vi "PT 100 Spannung zu Temp (SubVI).vi"(2 "Temp PT 100 soll":dbl, 3 "U ist 2":fxp<+/-,16,4>) -> (0 "U soll":fxp<+/-,16,4> format="%.14g", 1 "Temp PT 100 ist":dbl)   [LabVIEW 2010]
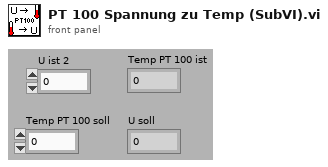
[diagram p1: front panel]
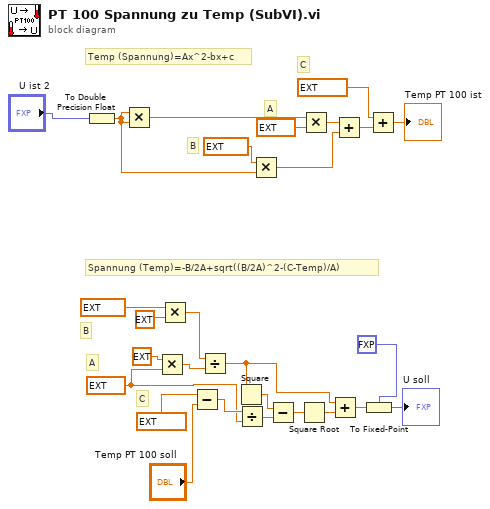
[diagram p0: block diagram]
diagram:
  w6 = ext 2.1471000000000000001 ("y")
  # "C"
  # "A"
  # "B"
  # "Spannung (Temp)=-B/2A+sqrt((B/2A)^2-(C-Temp)/A)"
  # "Temp (Spannung)=Ax^2-bx+c"
  # "C"
  # "A"
  # "B"
  n1 = To Double Precision Float(number="U ist 2") -> (double precision float=w1:dbl)
  n2 = Multiply(x=w1, y=w1) -> (x*y=w27:dbl)
  n3 = Multiply(x=ext 2.0 ("y"), y=w6) -> (x*y=w15:ext)
  n4 = Multiply(x=ext 111.873 ("y"), y=ext -1.0) -> (x*y=w17:ext)
  n5 = Subtract(x=ext -249.333 ("y"), y="Temp PT 100 soll") -> (x-y=w11:ext)
  n6 = Divide(x=w17, y=w15) -> (x/y=w8:ext)
  n7 = Square(x=w8) -> (x^2=w14:ext)
  n8 = Divide(x=w11, y=w6) -> (x/y=w10:ext)
  n9 = Multiply(x=ext 110.06300000000005 ("y"), y=w1) -> (x*y=w24:ext)
  n10 = Subtract(x=w14, y=w10) -> (x-y=w9:ext)
  n11 = Square Root(x=w9) -> (sqrt(x)=w7:ext)
  n12 = Multiply(x=w27, y=ext 2.1471 ("y 2")) -> (x*y=w23:ext)
  n13 = Add(x=w8, y=w7) -> (x+y=w5:ext)
  n14 = Add(x=w23, y=w24) -> (x+y=w22:ext)
  n15 = To Fixed-Point(fixed-point type=fxp<+/-,16,4> 0.0 ("Festkommatyp"), number=w5) -> (fixed-point=→"U soll":fxp<+/-,16,4>)
  n16 = Add(x=ext -249.333 ("y"), y=w22) -> (x+y=→"Temp PT 100 ist":ext)
